vi "TaskType.vi"() -> (1 "LinearConfig":T1={"decoding type"=10092, "units"=10219, "distance per pulse"=0.001, "initial position"=0.0, "z index enable"=FALSE, "z index value"=0.0, "z index phase"=10040, "CI_Encoder_A_InputTerm"="", "CI_Encoder_B_InputTerm"="", "CI_Encoder_Z_InputTerm"=""} {"units" items=["Meters"=10219, "Inches"=10379, "Ticks"=10304, "From Custom Scale"=10065]; "decoding type" items=["X1"=10090, "X2"=10091, "X4"=10092, "Two Pulse Counting"=10313]; "z index phase" items=["A High B High"=10040, "A High B Low"=10041, "A Low B High"=10042, "A Low B Low"=10043]}, 2 "AngularConfig":T2={"decoding type"=10092, "units"=10146, "pulses per revolution"=24, "initial angle"=0.0, "z index enable"=FALSE, "z index value"=0.0, "z index phase"=10040, "CI_Encoder_A_InputTerm"="", "CI_Encoder_B_InputTerm"="", "CI_Encoder_Z_InputTerm"=""} {"units" items=["Degrees"=10146, "Radians"=10273, "Ticks"=10304, "From Custom Scale"=10065]; "decoding type" items=["X1"=10090, "X2"=10091, "X4"=10092, "Two Pulse Counting"=10313]; "z index phase" items=["A High B High"=10040, "A High B Low"=10041, "A Low B High"=10042, "A Low B Low"=10043]}, 3 "AI_Config":T3={"AI"={"MaxValue"=10.0, "MinValue"=-10.0, "InputTerminalConfiguration"=10083}, "Scale"={"Offset"=0.0, "Gain"=1.0, "Unit"=""}, "Calibrate"={"K"=0.0, "B"=1.0}} {"AI"."InputTerminalConfiguration" items=["default"=-1, "RSE"=10083, "NRSE"=10078, "Differential"=10106, "Pseudodifferential"=12529]})   [LabVIEW 2025, in "DAQ_API.lvlib"]
uses:
  DAQ_API.lvlib
  DAQ_Module/DAQ_Module/DAQ_Module/DAQ_AI_Task_Config.ctl
  DAQ_Module/DAQ_Module/DAQ_Module/DAQ_Module.lvclass
  DAQ_Module/DAQ_Module/DAQ_Module/DAQ_Angular_Task_Config.ctl
  DAQ_Module/DAQ_Module/DAQ_Module/DAQ_Linear_Task_Config.ctl
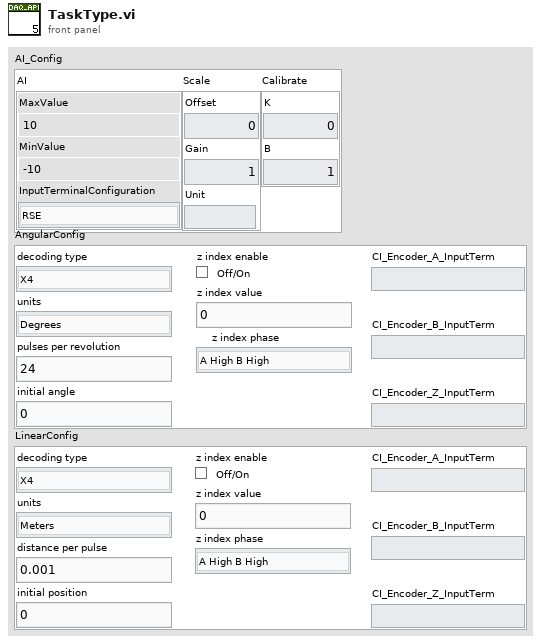
[diagram p1: front panel]
types:
  T1 = typedef "DAQ_Module.lvlib/DAQ_Module.lvclass/DAQ_Linear_Task_Config.ctl" = cluster{"decoding type":i32, "units":i32, "distance per pulse":dbl, "initial position":dbl, "z index enable":bool, "z index value":dbl, "z index phase":i32, "CI_Encoder_A_InputTerm":string, "CI_Encoder_B_InputTerm":string, "CI_Encoder_Z_InputTerm":string}
  T2 = typedef "DAQ_Module.lvlib/DAQ_Module.lvclass/DAQ_Angular_Task_Config.ctl" = cluster{"decoding type":i32, "units":i32, "pulses per revolution":u32, "initial angle":dbl, "z index enable":bool, "z index value":dbl, "z index phase":i32, "CI_Encoder_A_InputTerm":string, "CI_Encoder_B_InputTerm":string, "CI_Encoder_Z_InputTerm":string}
  T3 = typedef "DAQ_Module.lvlib/DAQ_Module.lvclass/DAQ_AI_Task_Config.ctl" = cluster{"AI":cluster{"MaxValue":dbl, "MinValue":dbl, "InputTerminalConfiguration":i32}, "Scale":cluster{"Offset":dbl, "Gain":dbl, "Unit":string}, "Calibrate":cluster{"K":dbl, "B":dbl}}
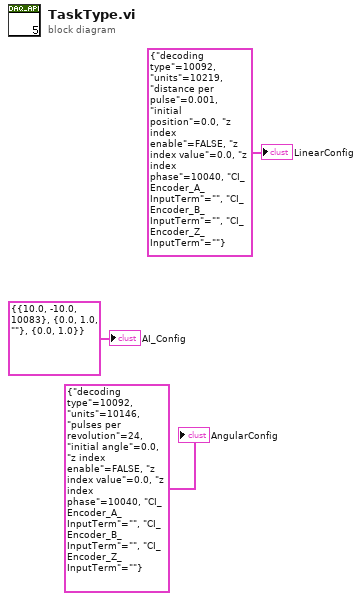
[diagram p0: block diagram]
diagram:
  "AI_Config" <- T3 {"AI"={"MaxValue"=10.0, "MinValue"=-10.0, "InputTerminalConfiguration"=10083}, "Scale"={"Offset"=0.0, "Gain"=1.0, "Unit"=""}, "Calibrate"={"K"=0.0, "B"=1.0}} ("AI_Config")
  "AngularConfig" <- T2 {"decoding type"=10092, "units"=10146, "pulses per revolution"=24, "initial angle"=0.0, "z index enable"=FALSE, "z index value"=0.0, "z index phase"=10040, "CI_Encoder_A_InputTerm"="", "CI_Encoder_B_InputTerm"="", "CI_Encoder_Z_InputTerm"=""} ("AngularConfig")
  "LinearConfig" <- T1 {"decoding type"=10092, "units"=10219, "distance per pulse"=0.001, "initial position"=0.0, "z index enable"=FALSE, "z index value"=0.0, "z index phase"=10040, "CI_Encoder_A_InputTerm"="", "CI_Encoder_B_InputTerm"="", "CI_Encoder_Z_InputTerm"=""} ("LinearConfig")
